vi "Stop Octave.vi"(6 "Stop Octave? (T)":bool=TRUE, 8 "error in (no error)":errorcluster) -> (0 "error out":errorcluster)   [LabVIEW 2020]
doc: "Stops Octave if input set to stop."
uses:
  external libraries/GOLPI 0.7.3.1 source distribution LV 20.0 32 bit/GOLPI reference Type Def.ctl
  external libraries/GOLPI 0.7.3.1 source distribution LV 20.0 32 bit/Pipe Handle.ctl
  Globals for GOLPI.vi
  external libraries/GOLPI 0.7.3.1 source distribution LV 20.0 32 bit/LV Process library.lvlib
  external libraries/GOLPI 0.7.3.1 source distribution LV 20.0 32 bit/GOLPI library.lvlib
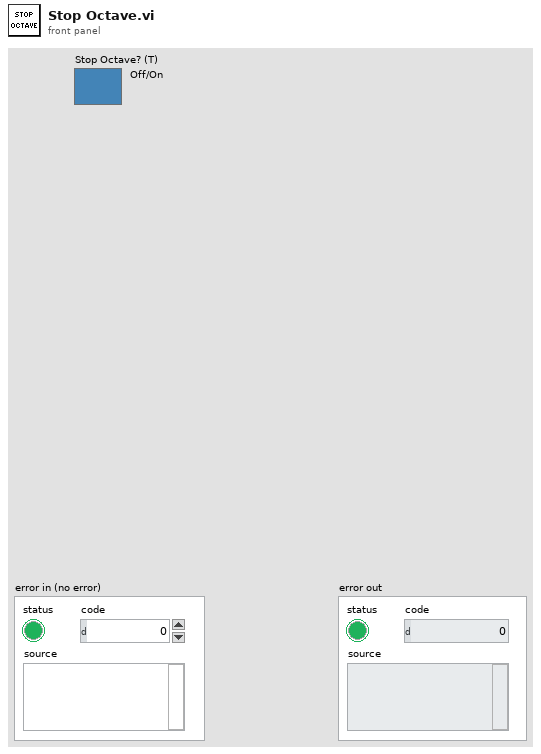
[diagram p1: front panel]
types:
  T1 = typedef "GOLPI library.lvlib/GOLPI reference Type Def.ctl" = cluster{"pipe handle":T2, "fast read timeout [ms]":u32, "fast read settle time [ms]":u32, "fast read to multiple [ms]":u32, "max elements per input line":u32, "slow read timeout [ms]":u32, "stdin double format specifier":string, "max elements per stdout output column":u32, "console mode bitstream":bool, "bitstream first read timeout [ms]":u32, "bitstream read timeout [ms]":u32, "struct transfer possible":bool, "matlab mode":bool}
  T2 = typedef "LV Process library.lvlib/Pipe Handle.ctl" = cluster{"lv_proc.dll file path":path, "process instance handle":u32[], "debug mode":bool, "debug data":cluster{"time":timestamp, "stdin":bool, "data":string}[]}
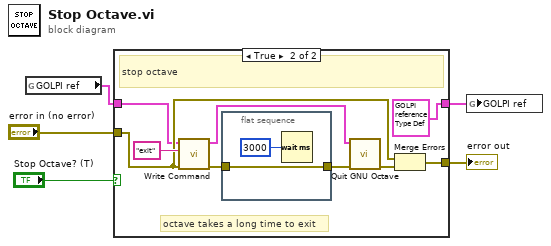
[diagram p0: block diagram]
diagram:
  n1 = global read "Globals for GOLPI.vi" "GOLPI ref"() -> (w2:T1)
  n2 = case shown="True" "Stop Octave? (T)" {
    tunnel: [w7 w14] -> w3
    tunnel: "error in (no error)" -> [w7 w12]
    tunnel: w2 -> [w6 w11]
    tunnel: [w6 T1 {"pipe handle"={"lv_proc.dll file path"=path "", "process instance handle"=[], "debug mode"=FALSE, "debug data"=[]}, "fast read timeout [ms]"=500, "fast read settle time [ms]"=10, "fast read to multiple [ms]"=1, "max elements per input line"=100, "slow read timeout [ms]"=5000, "stdin double format specifier"="%_16e", "max elements per stdout output column"=100, "console mode bitstream"=FALSE, "bitstream first read timeout [ms]"=1000, "bitstream read timeout [ms]"=50, "struct transfer possible"=FALSE, "matlab mode"=FALSE} ("GOLPI ref. out")] -> w1
    frame False {
    }
    frame True {
      # "octave takes a long time to exit"
      # "stop octave"
      n3 = call "Write Command.vi"("error in"=w12, "command"="exit", "GOLPI ref. in"=w11) -> ("error out"=w8:errorcluster, "GOLPI ref. out"=w10:T1)  [unwired: 7 in]
      n4 = flat-sequence {
        tunnel: [w17] -> w9
        tunnel: w8 -> [w17]
        frame #0 {
          n5 = Wait (ms)(milliseconds to wait=u32 3000) -> ()  [unwired: 1 out]
        }
      }
      n6 = call "Quit GNU Octave.vi"("error in"=w9, "GOLPI ref. in"=w10) -> ("error out"=w15:errorcluster)  [unwired: 8 in, 1 out]
      n7 = Merge Errors(w12, w15) -> (w14:errorcluster)
    }
  }
  "error out" <- w3
  n8 = global write "Globals for GOLPI.vi" "GOLPI ref"(w1) -> ()
